vi "Launch TDMS File Viewer.vi"() -> ()   [LabVIEW 2017]
doc: "Developed by Kevin Thompson\nkevin@thompsonengineering.net\n\nCopyright 2018-2020\nThompson Engineering, LLC"
panel:
  in  "Quit":bool
  in  "ViewTDMS":bool
  # "TDMS File Viewer"
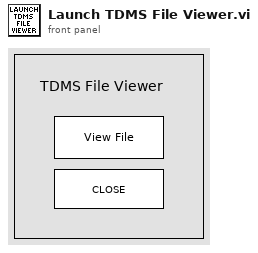
[diagram p1: front panel]
types:
  T1 = enum32{"Invalid", "Standard", "Closed", "Hidden", "Minimized", "Maximized"}
  T2 = typedef "TD Pathnames--cluster.ctl" = cluster{"RunTimeSys?":bool, "AppFolder":path, "ExecutablePath":path, "ConfigFolder":path, "DataLogFolder":path, "SystemLogFolder":path, "SeqFolder":path, "MainStartupPathname":path, "MainUIPathname":path, "SystemEventsFile":path, "SeqEventsFile":path, "Config SettingsFile":path, "DAQ IOConfigFile":path, "SystemSimulation":bool}
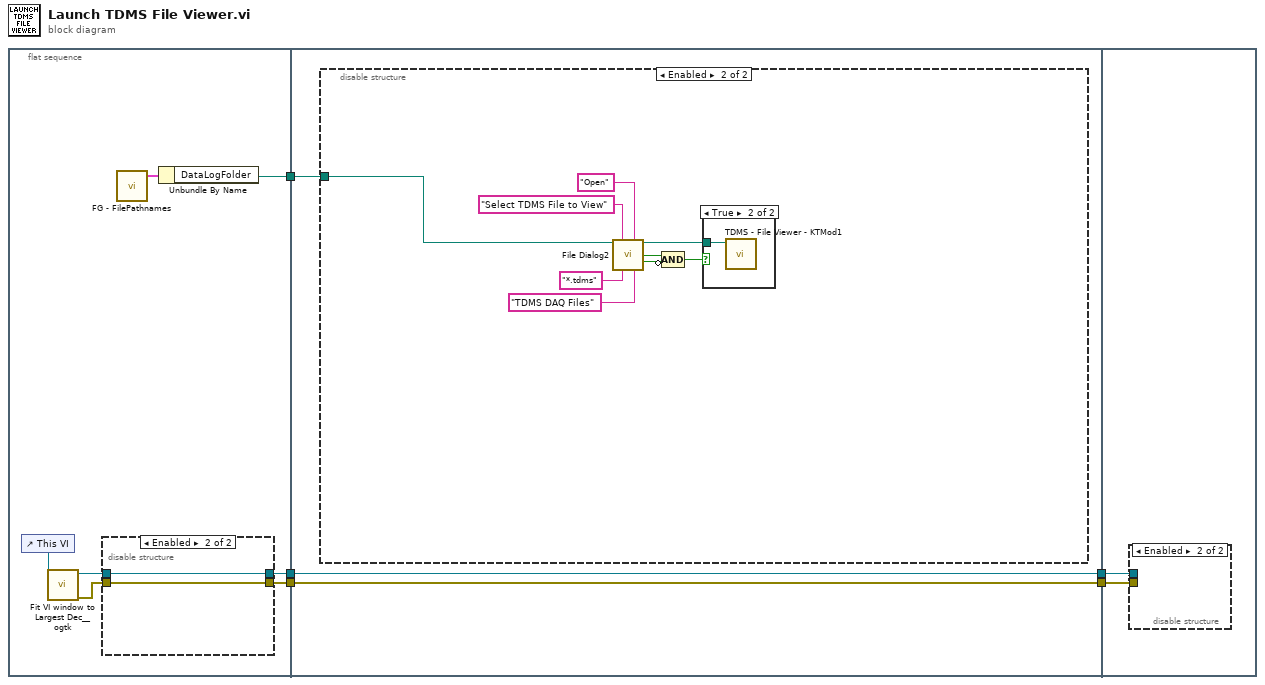
[diagram p0: block diagram]
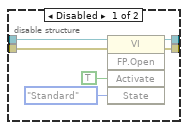
[diagram p2: hidden frame]
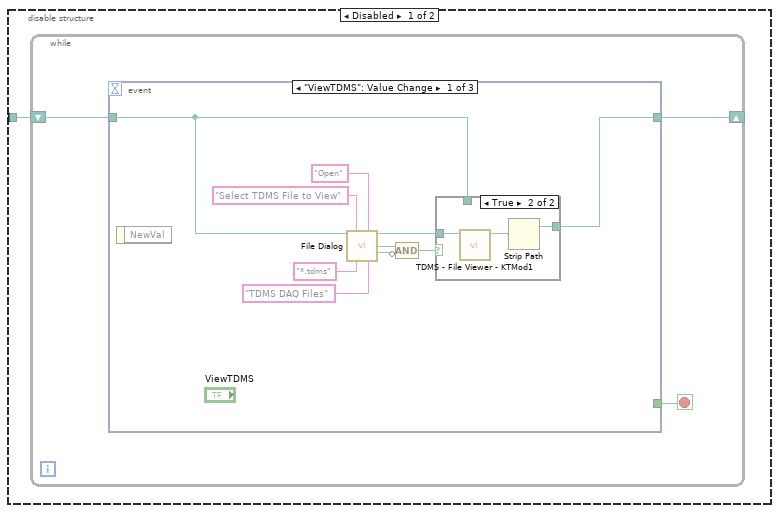
[diagram p3: hidden frame]
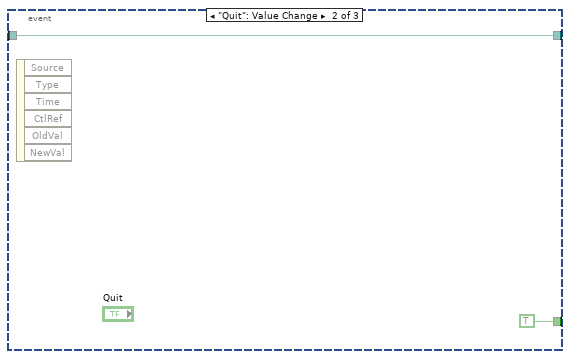
[diagram p5: hidden frame]
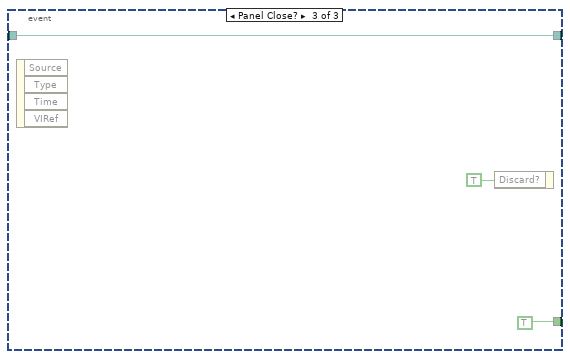
[diagram p6: hidden frame]
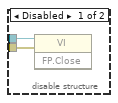
[diagram p8: hidden frame]
diagram:
  n1 = flat-sequence {
    tunnel: [w6] -> w5
    tunnel: [w11] -> w4
    tunnel: [w8] -> w2
    tunnel: w5 -> [w23]
    tunnel: w4 -> [w22]
    tunnel: [w22] -> w3
    tunnel: w2 -> [w21]
    tunnel: [w21] -> w1
    tunnel: w3 -> [w58]
    tunnel: w1 -> [w57]
    frame #0 {
      n2 = control-ref of="This VI"() -> (w10:refnum<vi>)
      n3 = call <userlib>:"Fit VI window to Largest Dec__ogtk.vi"("VI Ref (calling VI)"=w10) -> ("error out"=w9:errorcluster, "dup VI Ref"=w12:refnum<vi>)  [unwired: 5 in]
      n4 = disable-structure shown="Enabled" {
        disable-tunnel: w12 -> [w18 w19]
        disable-tunnel: [w15 w19] -> w11
        disable-tunnel: w9 -> [w14 w20]
        disable-tunnel: [w13 w20] -> w8
        frame Disabled {
          n5 = invoke class="VI" method="FP.Open"(reference=w18, error in=w14, "Activate"=TRUE ("Activate?"), "State"=T1."Standard") -> (reference out=w15:refnum<vi>, error out=w13:errorcluster)  [unwired: 1 in, 3 out]
        }
        frame Enabled {
        }
      }
      n6 = call "FG - FilePathnames.vi"() -> ("FilePaths out"=w7:T2)  [unwired: 4 in, 1 out]
      n7 = Unbundle By Name(w7) -> ("DataLogFolder"=w6:path)
    }
    frame #1 {
      n8 = disable-structure shown="Enabled" {
        disable-tunnel: w23 -> [w24 w48]
        frame Disabled {
          n9 = while {
            shift-right: [w25] -> _
            shift-left: w24 -> [w26]
            stop <- w27 stop-if-true
            n10 = event shown="[0] \"ViewTDMS\": Value Change" {
              selector: _ -> [_ _ _]
              dyn-events: _ -> [_ _ _]
              timeout: _ -> [_ _ _]
              tunnel: [_ TRUE TRUE] -> w27
              tunnel: w26 -> [w29 w42 w44]
              tunnel: [w28 w42 w44] -> w25
              event "ViewTDMS": Value Change {
                n11 = event-data() -> ()  [unwired: 1 in, 1 out]
                n12 = call "File Dialog"("start path"=w29, "prompt"="Select TDMS File to View", "button label"="Open", "pattern (all files)"="*.tdms", "pattern label"="TDMS DAQ Files") -> ("selected path"=w33:path, "exists"=w32:bool, "cancelled"=w31:bool)  [unwired: 7 in, 1 out]
                n13 = Compound Arithmetic op=AND(w32, invert w31) -> (w30:bool)
                n14 = case shown="True" w30 {
                  tunnel: w33 -> [_ w41]
                  tunnel: w29 -> [w38 _]
                  tunnel: [w38 w39] -> w28
                  frame False {
                  }
                  frame True {
                    n15 = call "TDMS - File Viewer - KTMod1.vi"("file path"=w41) -> ("file path out"=w40:path)  [unwired: 5 in, 1 out]
                    n16 = Strip Path(path=w40) -> (stripped path=w39:path)  [unwired: 1 out]
                  }
                }
              }
              event "Quit": Value Change {
                n17 = event-data() -> ()  [unwired: 1 in, 6 out]
              }
              event Panel Close? {
                n18 = event-data() -> ()  [unwired: 1 in, 4 out]
                n19 = event-data("Discard?"=TRUE) -> ()  [unwired: 1 in, 1 out]
              }
            }
          }
        }
        frame Enabled {
          n20 = call "File Dialog2"("start path"=w48, "prompt"="Select TDMS File to View", "button label"="Open", "pattern (all files)"="*.tdms", "pattern label"="TDMS DAQ Files") -> ("selected path"=w55:path, "exists"=w54:bool, "cancelled"=w53:bool)  [unwired: 7 in, 1 out]
          n21 = Compound Arithmetic op=AND(w54, invert w53) -> (w47:bool)
          n22 = case shown="True" w47 {
            tunnel: w55 -> [_ w56]
            frame False {
            }
            frame True {
              n23 = call "TDMS - File Viewer - KTMod1.vi"("file path"=w56) -> ()  [unwired: 5 in, 2 out]
            }
          }
        }
      }
    }
    frame #2 {
      n24 = disable-structure shown="Enabled" {
        disable-tunnel: w58 -> [w60 _]
        disable-tunnel: w57 -> [w59 _]
        frame Disabled {
          n25 = invoke class="VI" method="FP.Close"(reference=w60, error in=w59) -> ()  [unwired: 1 in, 3 out]
        }
        frame Enabled {
        }
      }
    }
  }
